vi "System@RecordCycleTime__Parameter.vi"(1 "ParamterIn":string) -> (0 "ParamterOut":string)   [LabVIEW 2020]
panel:
  in  "Message2":string(combo)
  in  "Message1":string(combo)
  in  "Record":string(combo)
  in  "Confirm":bool
  # "System@RecordCycleTime $Record,$Message1(,$Message2)"
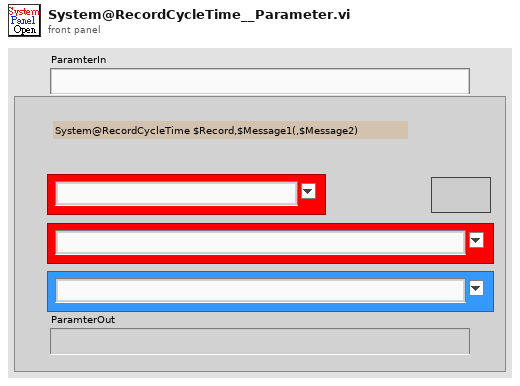
[diagram p1: front panel]
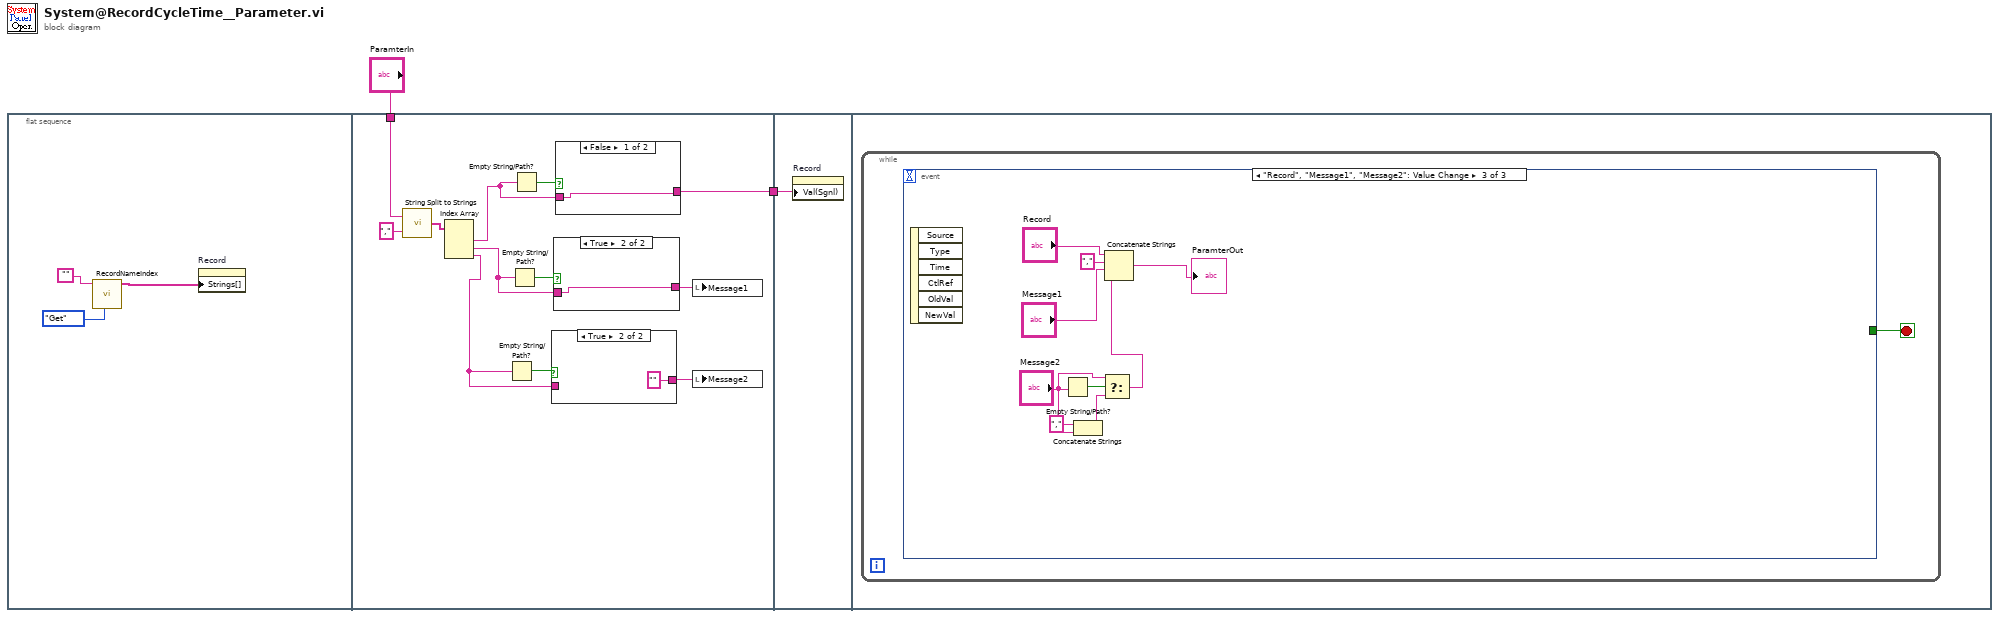
[diagram p0: block diagram]
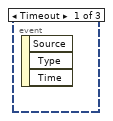
[diagram p5: hidden frame]
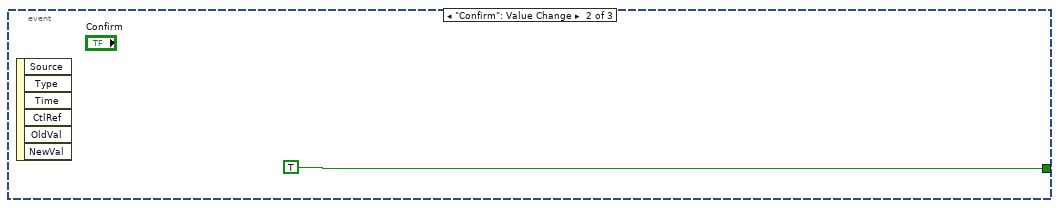
[diagram p6: hidden frame]
diagram:
  n1 = flat-sequence {
    tunnel: "ParamterIn" -> [w11]
    tunnel: [w15] -> w1
    tunnel: w1 -> [w24]
    frame #0 {
      n2 = call "RecordNameIndex.vi"("OP"=enum16{"Init", "Insert", "Get", "Write", "Read"}."Get", "ItemCatalog"="") -> ("NamelList"=w3:string[])  [unwired: 6 in, 3 out]
      n3 = property on="Record" class="CmbBox"("Strings[]"=w3) -> ()  [unwired: 2 in, 2 out]
    }
    frame #1 {
      n4 = call "String Split to Strings.vi"("search string/char (-)"=",", "String"=w11) -> ("Array"=w9:string[])
      n5 = Index Array(array=w9) -> (element #1=w8:string, element #2=w7:string, element #3=w6:string)  [unwired: 3 in]
      n6 = Empty String/Path?(string/path=w6) -> (empty?=w13:bool)
      n7 = Empty String/Path?(string/path=w7) -> (empty?=w16:bool)
      n8 = Empty String/Path?(string/path=w8) -> (empty?=w17:bool)
      n9 = case shown="True" w13 {
        tunnel: w6 -> [w18 _]
        tunnel: [w18 "" ("ParamterIn")] -> w12
        frame False {
        }
        frame True {
        }
      }
      n10 = case shown="True" w16 {
        tunnel: w7 -> [w20 w21]
        tunnel: [w20 w21] -> w14
        frame False {
        }
        frame True {
        }
      }
      n11 = case shown="False" w17 {
        tunnel: w8 -> [w22 w23]
        tunnel: [w22 w23] -> w15
        frame False {
        }
        frame True {
        }
      }
      n12 = local write "Message1"(w14) -> ()
      n13 = local write "Message2"(w12) -> ()
    }
    frame #2 {
      n14 = property on="Record" class="CmbBox"("Val(Sgnl)"=w24) -> ()  [unwired: 2 in, 2 out]
    }
    frame #3 {
      n15 = while {
        stop <- w25 stop-if-true
        n16 = event shown="[2] \"Record\", \"Message1\", \"Message2\": Value Change" {
          selector: _ -> [_ _ _]
          dyn-events: _ -> [_ _ _]
          timeout: _ -> [_ _ _]
          tunnel: [_ TRUE _] -> w25
          event Timeout {
            n17 = event-data() -> ()  [unwired: 1 in, 3 out]
          }
          event "Confirm": Value Change {
            n18 = event-data() -> ()  [unwired: 1 in, 6 out]
          }
          event "Record", "Message1", "Message2": Value Change {
            n19 = event-data() -> ()  [unwired: 1 in, 6 out]
            n20 = Empty String/Path?(string/path="Message2") -> (empty?=w31:bool)
            n21 = Concatenate Strings("," ("string"), "Message2") -> (w28:string)
            n22 = Select(t="Message2", s=w31, f=w28) -> (s? t:f=w27:string)
            n23 = Concatenate Strings("Record", "," ("string"), "Message1", w27) -> (→"ParamterOut":string)
          }
        }
      }
    }
  }
